vi "Wait_Cycle_Over.vi"(6 "Standalone?":bool, 8 "Error In":errorcluster, 9 "GEA2 Reference In":refnum<k24>, 10 "GEA Inputs":T1 {"Destination" format="%.0x"; "Source" format="%.0x"}, 11 "Device Selected":i32) -> (0 "Error Out":errorcluster, 1 "GEA2 Reference Out":refnum<k24>, 3 "Cycle Complete":bool)   [LabVIEW 2014]
uses:
  Common/LabVIEW GEA2 Toolkit/LabVIEW_GEA2_Toolkit.lvlibp/type defs/Source_Destination.ctl
  Common/LabVIEW GEA2 Toolkit/LabVIEW_GEA2_Toolkit.lvlibp/type defs/ERD Read Data In.ctl
  Common/LabVIEW GEA2 Toolkit/LabVIEW_GEA2_Toolkit.lvlibp/type defs/Data Type.ctl
  Common/LabVIEW GEA2 Toolkit/LabVIEW_GEA2_Toolkit.lvlibp
  C:/Automation/DLLs/PC Tools .NET/GeaCommunication.dll
panel:
  out "Heartbeat":bool
  out "Status 2000":string
  # "Poll ERD 2000 every 2 sec.\nExit on EOC (4) or Idle State (0)."
  # "Changes state every 2 sec.\nwhile VI is running."
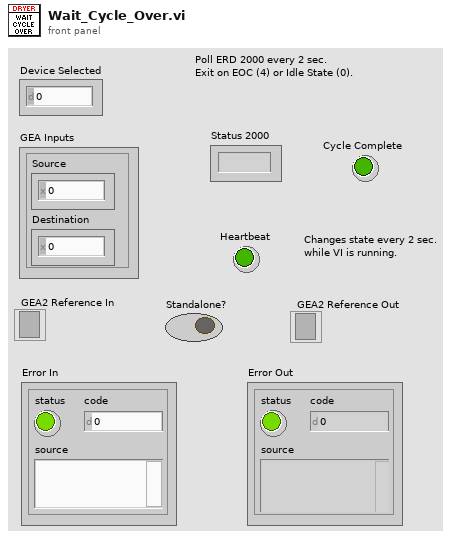
[diagram p1: front panel]
types:
  T1 = typedef "LabVIEW_GEA2_Toolkit.lvlibp/Source_Destination.ctl" = cluster{"Source":u8, "Destination":u8}
  T2 = typedef "LabVIEW_GEA2_Toolkit.lvlibp/ERD Read Data In.ctl" = cluster{"ERD Number":u16, "Data Type":T3}
  T3 = typedef "LabVIEW_GEA2_Toolkit.lvlibp/Data Type.ctl" = enum16{"string", "boolean", "uint8_t", "uint16_t", "uint32_t", "uint64_t", "int8_t", "int16_t", "int32_t", "int64_t"}
  T4 = typedef "LabVIEW_GEA2_Toolkit.lvlibp/ERD Read Data Out.ctl" = cluster{"ERD Number":u16, "Data":string}
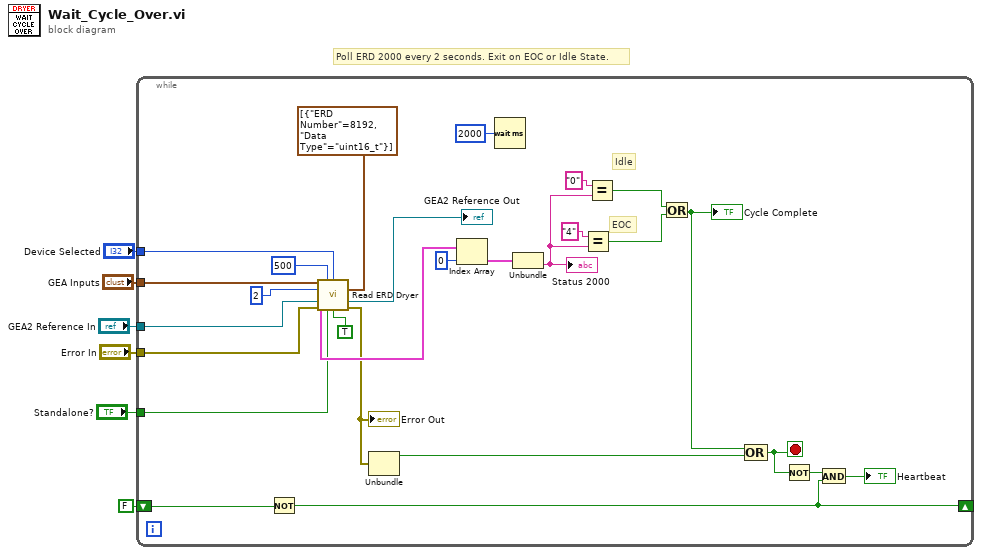
[diagram p0: block diagram]
diagram:
  # "Poll ERD 2000 every 2 seconds. Exit on EOC or Idle State."
  n1 = while {
    tunnel: "GEA Inputs" -> [w33]
    tunnel: "Device Selected" -> [w32]
    tunnel: "Error In" -> [w22]
    shift-right: [w17] -> _
    shift-left: FALSE -> [w20]
    tunnel: "Standalone?" -> [w14]
    tunnel: "GEA2 Reference In" -> [w13]
    stop <- w19 stop-if-true
    # "Idle"
    # "EOC"
    n2 = Not(x=w20) -> (.not. x?=w17:bool)
    n3 = call "Read ERD Dryer.vi"("GEA Inputs"=w33, "Read Timeout (ms)"=u32 500, "Device Selected"=w32, "Retry Count"=2, "Read ERD List"=T2[] [{"ERD Number"=8192, "Data Type"=enum."uint16_t"}], "GEA2 Reference In"=w13, "Error In"=w22, "Standalone?"=w14, "Verify ERD Response?"=TRUE) -> ("ERD Data Out"=w27:T4[], "GEA2 Reference Out"=→"GEA2 Reference Out":refnum<k24>, "Error Out"=w23:errorcluster)  [unwired: 3 in, 1 out]
    "Error Out" <- w23
    n4 = Unbundle(w23) -> ("status"=w12:bool)  [unwired: 2 out]
    n5 = Index Array(array=w27, index=0) -> (element=w25:T4)
    n6 = Wait (ms)(milliseconds to wait=u32 2000) -> ()  [unwired: 1 out]
    n7 = Unbundle(w25) -> ("Data"=w10:string)  [unwired: 1 out]
    "Status 2000" <- w10
    n8 = Equal?(x="4", y=w10) -> (x = y?=w7:bool)
    n9 = Equal?(x="0", y=w10) -> (x = y?=w8:bool)
    n10 = Or(x=w8, y=w7) -> (x .or. y?=w9:bool)
    "Cycle Complete" <- w9
    n11 = Compound Arithmetic op=OR(w9, w12) -> (w19:bool)
    n12 = Not(x=w19) -> (.not. x?=w18:bool)
    n13 = And(x=w18, y=w17) -> (x .and. y?=→"Heartbeat":bool)
  }
